vi "Close Library.vi"(8 "error in (no error)":errorcluster) -> (0 "error out":errorcluster)   [LabVIEW 2016, in "Hall Effect Library.lvlib"]
uses:
  Hall Effect Library.lvlib
  Private/Global Variables/Communication.vi
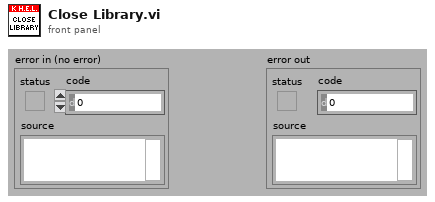
[diagram p1: front panel]
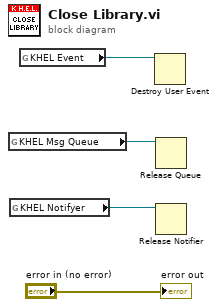
[diagram p0: block diagram]
diagram:
  n1 = global read "Communication.vi" "KHEL Msg Queue"() -> (w4:refnum<queue>)
  n2 = global read "Communication.vi" "KHEL Notifyer"() -> (w3:refnum<notifier>)
  n3 = global read "Communication.vi" "KHEL Event"() -> (w1:refnum<user-event>)
  n4 = Destroy User Event(user event=w1) -> ()  [unwired: 1 in, 1 out]
  n5 = Release Queue(queue=w4) -> ()  [unwired: 1 in, 4 out]
  n6 = Release Notifier(notifier=w3) -> ()  [unwired: 1 in, 4 out]
  "error out" <- "error in (no error)"
